vi "Constructor_SQLiteLogHandle.vi"(7 "TableName (event_log)":string="event_log", 8 "error in (no error)":errorcluster, 10 "db file":path) -> (0 "error out":errorcluster, 3 "SQLiteLogHandle out":refnum<class "SQLiteLogHandle.lvclass">)   [LabVIEW 2024, in "SQLiteLogHandle.lvclass"]
uses:
  SQLiteLogHandle.lvclass
  SQLiteLogHandle.lvclass/SQLiteLogHandle.ctl
  <vilib>/drjdpowell/SQLite Library/SQL Connection/Connection.lvclass
  <vilib>/drjdpowell/SQLite Library/SQL Connection/Open (path).vi
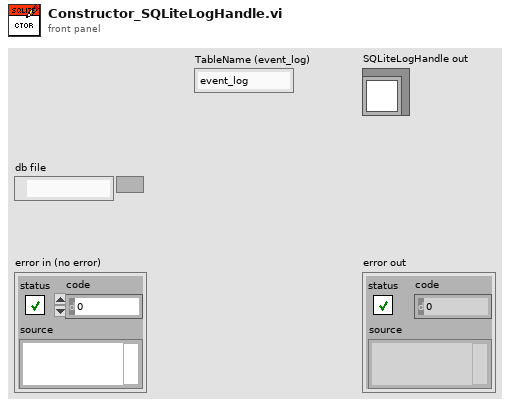
[diagram p1: front panel]
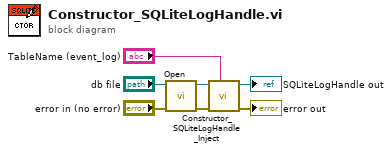
[diagram p0: block diagram]
diagram:
  n1 = call-poly <vilib>:"Open.vi"("error in (no error)"="error in (no error)", "db file"="db file") -> ("error out"=w3:errorcluster, "SQLite Connection"=w2:refnum<class "Connection.lvclass">)  [unwired: 8 in]
  n2 = call "Constructor_SQLiteLogHandle_Inject.vi"("TableName (event_log)"="TableName (event_log)", "error in (no error)"=w3, "Connection in"=w2) -> ("error out"=→"error out":errorcluster, "SQLiteLogHandle out"=→"SQLiteLogHandle out":refnum<class "SQLiteLogHandle.lvclass">)  [unwired: 7 in]
